vi "Build Tree From Classes.vi"(5 "Selected Item (None)":string, 6 "Close Items":bool, 7 "Show":T2={"Show Private"=TRUE, "Show Scripting"=FALSE}, 8 "error in":errorcluster, 9 "Filter":string, 10 "Class Tree Array":T1[](array[typedef]), 11 "Tree Ref":refnum<vi>) -> (0 "error out":errorcluster, 3 "Tree Ref Out":refnum<vi>)   [LabVIEW 2023]
doc: "Take a cluster reference and build a tree of all items in cluster. Set tags of items as \"[row number] item name\" so all tags are unique. Set glyph of its to indicate data type. Set selection color to gray and font size to 18pt."
uses:
  class/Class Item Cluster.ctl
  <userlib>/_OpenG.lib/comparison/comparison.llb/Variant Changed__ogtk.vi
panel:
  out "exe time (ms)":u32
  in  "Tree":string[](tree)
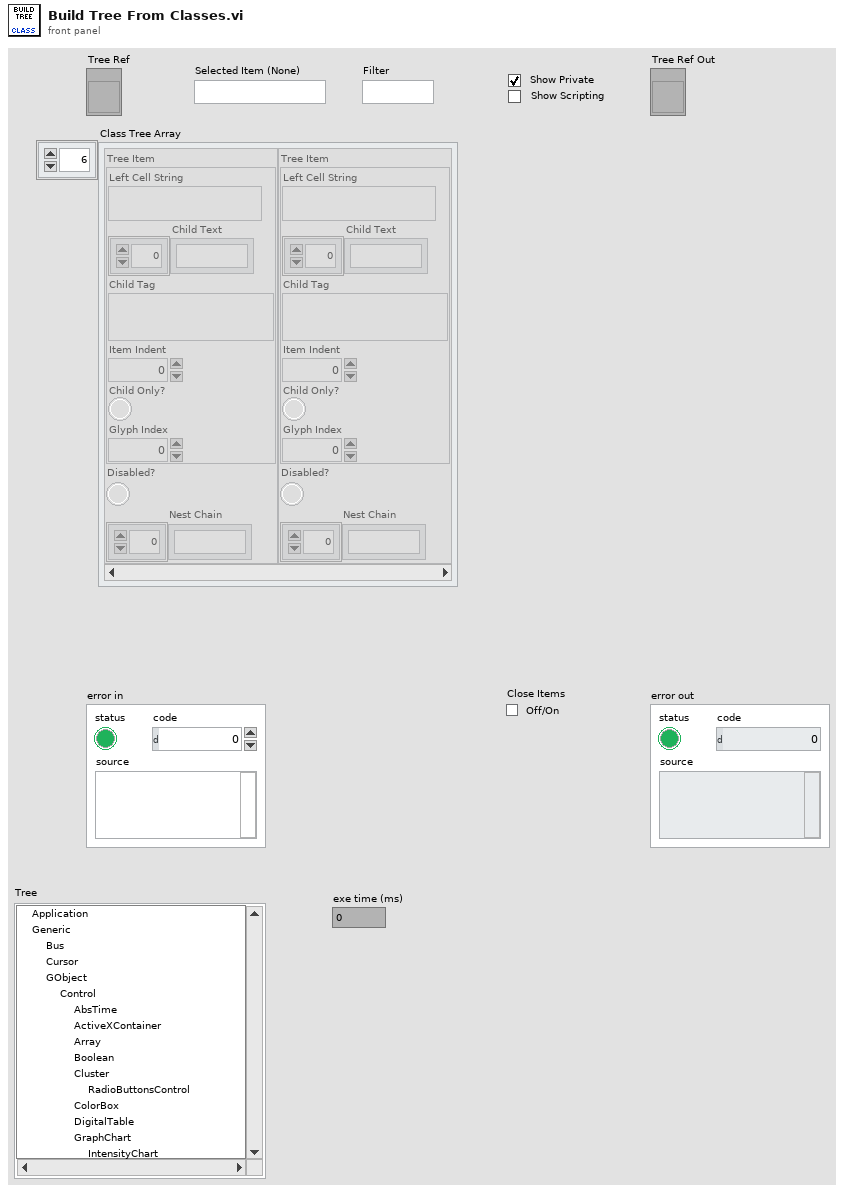
[diagram p1: front panel]
types:
  T1 = typedef "Class Item Cluster.ctl" = cluster{"Tree Item":cluster{"Left Cell String":string, "Child Text":string[], "Child Tag":string, "Item Indent":i32, "Child Only?":bool, "Glyph Index":i32}, "Disabled?":bool, "Nest Chain":string[]}
  T2 = cluster{"Show Private":bool, "Show Scripting":bool}
  T3 = cluster{"Left Cell String":string, "Child Text":string[], "Child Tag":string, "Item Indent":i32, "Child Only?":bool, "Glyph Index":i32}[]
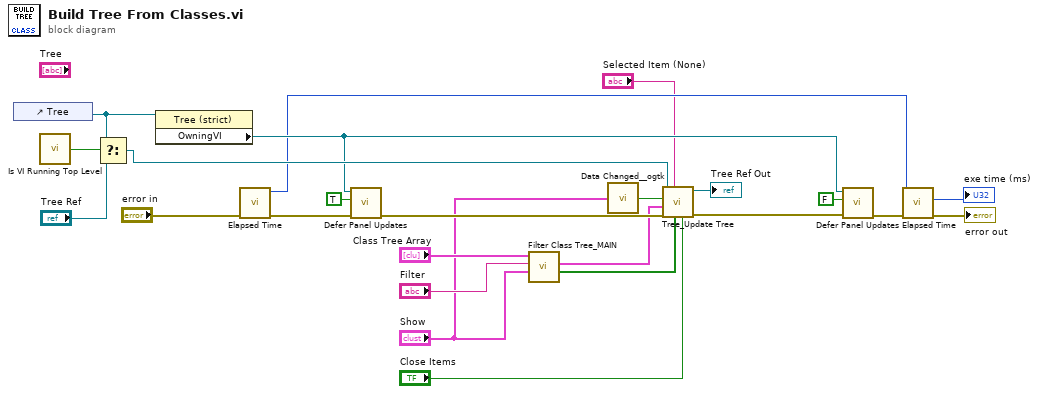
[diagram p0: block diagram]
diagram:
  n1 = control-ref of="Tree"() -> (w18:refnum<vi>)
  n2 = call "Is VI Running Top Level.vi"() -> ("Top Level?"=w24:bool)  [unwired: 5 in]
  n3 = Select(t=w18, s=w24, f="Tree Ref") -> (s? t:f=w22:refnum<vi>)
  n4 = property class="Tree (strict)"(reference=w18) -> ("OwningVI"=w17:refnum<vi>)  [unwired: 1 in, 2 out]
  n5 = call "Elapsed Time.vi"("error in"="error in") -> ("error out"=w14:errorcluster, "millisecond timer value"=w9:u32)  [unwired: 6 in, 3 out]
  n6 = call "Defer Panel Updates.vi"("error in (no error)"=w14, "Defer Panel Updates [T]"=TRUE, "VI Ref"=w17) -> ("error out"=w21:errorcluster)  [unwired: 7 in, 1 out]
  n7 = call "Filter Class Tree_MAIN.vi"("Show"="Show", "Filter"="Filter", "Class Items In"="Class Tree Array") -> ("Disabled?"=w5:bool[], "Class Tree Arr"=w8:T3)  [unwired: 6 in, 1 out]
  n8 = call-poly <userlib>:"Data Changed__ogtk.vi"("Variant"="Show") -> ("Changed"=w6:bool)
  n9 = call "Tree_Update Tree.vi"("Close Items"="Close Items", "Disabled?"=w5, "Focus Item"="Selected Item (None)", "error in"=w21, "New Items"=w8, "Show Changed"=w6, "TreeControl in"=w22) -> ("error out"=w3:errorcluster, "TreeControl out"=→"Tree Ref Out":refnum<vi>)  [unwired: 3 in]
  n10 = call "Defer Panel Updates.vi"("error in (no error)"=w3, "Defer Panel Updates [T]"=FALSE, "VI Ref"=w17) -> ("error out"=w13:errorcluster)  [unwired: 7 in, 1 out]
  n11 = call "Elapsed Time.vi"("error in"=w13, "past time"=w9) -> ("error out"=→"error out":errorcluster, "elapsed time (ms)"=→"exe time (ms)":u32)  [unwired: 5 in, 3 out]
